vi "FTW-JSON-Object-Join-String.vi"(0 "JSON":T2, 5 "JSON String to Join":string, 7 "Update Mode":T1, 11 "error in":errorcluster) -> (4 "JSON out":T2, 15 "error out":errorcluster)   [LabVIEW 2015]
uses:
  core/type/FTW-Type-JSON.ctl
  FTW-JSON-JoinMode.ctl
panel:
  # "Inputs"
  # "Outputs"
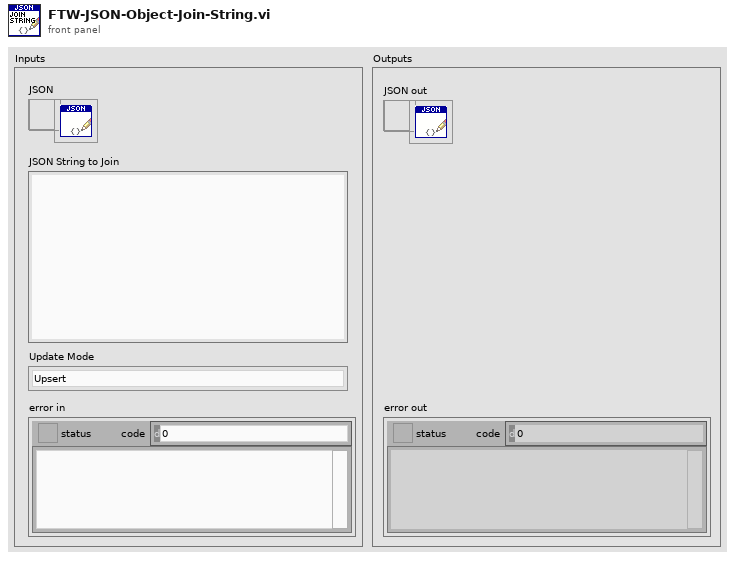
[diagram p1: front panel]
types:
  T1 = typedef "FTW-JSON-JoinMode.ctl" = enum32{"Upsert", "Update Only", "Insert Only"}
  T2 = typedef "FTW-Type-JSON.ctl" = refnum<data-value>
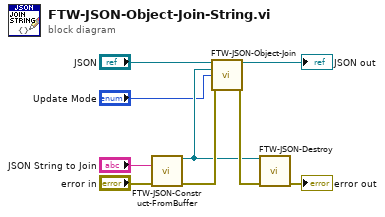
[diagram p0: block diagram]
diagram:
  n1 = call "FTW-JSON-Construct-FromBuffer.vi"("JSON String (UTF-8)"="JSON String to Join", "error in"="error in") -> ("JSON"=w2:T2, "error out"=w4:errorcluster)  [unwired: 12 in]
  n2 = call "FTW-JSON-Object-Join.vi"("JSON"="JSON", "JSON to Join"=w2, "Join Mode"="Update Mode", "error in"=w4) -> ("JSON out"=→"JSON out":T2, "error out"=w3:errorcluster)  [unwired: 10 in]
  n3 = call "FTW-JSON-Destroy.vi"("JSON"=w2, "error in"=w3) -> ("error out"=→"error out":errorcluster)  [unwired: 13 in]
